vi "CALC_SMO_STAT_ON_OFF.vi"(0 "VISA IN":refnum<visa-resource-name>, 1 "Smoothing ON/OFF":bool, 5 "error in":errorcluster, 7 "Channel":i32) -> (14 "VISA Out":refnum<visa-resource-name>, 19 "error out":errorcluster)   [LabVIEW 2018, in "PNA-X.lvlib"]
doc: "CALCulate<cnum>:SMOothing[:STATe] <ON | OFF> \n(Read-Write) Turns data smoothing ON or OFF. \nSee Critical Note \nParameters \n<cnum> Channel number of the measurement. There must be a selected measurement \non that channel. If unspecified, <cnum> is set to 1. \n<ON | OFF> ON (or 1) - turns smoothing ON. \nOFF (or 0) - turns smoothing OFF. \nExamples CALC:SMO ON \ncalculate2:smoothing:state off \nQuery Syntax CALCulate<cnum>:SMOothing[:STATe]? \nReturn Type Boolean (1 = ON, 0 = OFF) \nDefault OFF \n1564\n\n1565\n\nCalculate:Transform Commands \nSpecifies the settings for time domain transform. \nClick on a blue keyword to view the command details. \nSee Also \nExample Programs \nLearn about Time Domain \nSynchronizing the PNA and Controller \nSCPI Command Tree \nCritical Note: CALCulate commands act on the selected measurement. You can select one \nmeasurement for each channel using Calc:Par:Select"
uses:
  PNA-X.lvlib
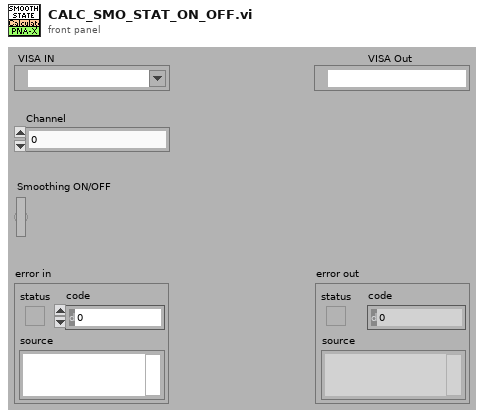
[diagram p1: front panel]
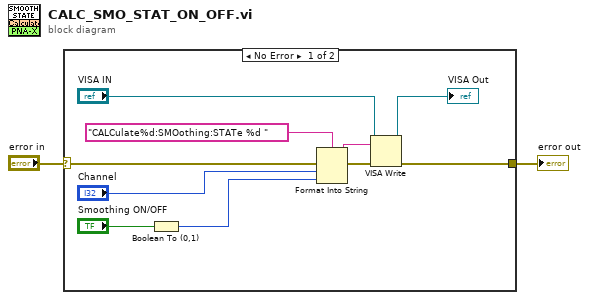
[diagram p0: block diagram]
diagram:
  n1 = case shown="No Error" "error in" {
    selector: "error in" -> [w12 w13]
    tunnel: [w7 w13] -> w1
    frame No Error {
      n2 = Boolean To (0,1)(Boolean="Smoothing ON/OFF") -> (0, 1=w3:i16)
      n3 = Format Into String(format string="CALCulate%d:SMOothing:STATe %d " ("Cmdline"), error in=w12, "Channel", w3) -> (resulting string=w10:string, error out=w11:errorcluster)  [unwired: 1 in]
      n4 = VISA Write(VISA resource name="VISA IN", write buffer=w10, error in (no error)=w11) -> (VISA resource name out=→"VISA Out":refnum<visa-resource-name>, error out=w7:errorcluster)  [unwired: 1 out]
    }
    frame Error {
    }
  }
  "error out" <- w1
